vi "Update.vi"(8 "error in (no error)":errorcluster, 9 "Operation":enum16{"Get", "Set"}(ring), 11 "user event":refnum<user-event>) -> (0 "error out":errorcluster, 3 "user event (out)":refnum<user-event>)   [LabVIEW 2020, in "WebServiceImporter.lvlib" / "Main Panel.lvlib" / "Authentication.lvlib" / "Events.lvlib"]
uses:
  <vilib>/Platform/WebService/Main Panel/Pages/Authentication/Events/Events.lvlib
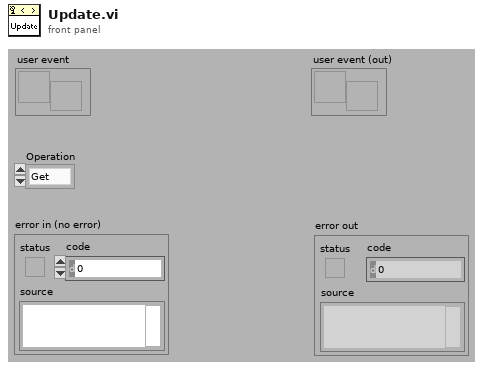
[diagram p1: front panel]
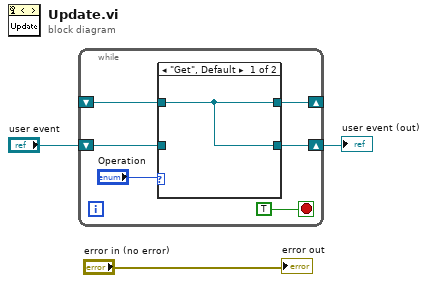
[diagram p0: block diagram]
diagram:
  n1 = while {
    shift-right: [w7] -> w1
    shift-left: "user event" -> [w8]
    shift-right: [w6] -> _
    shift-left: _ -> [w5]
    stop <- TRUE stop-if-true
    n2 = case shown="\"Get\", Default" "Operation" {
      tunnel: w8 -> [_ w11]
      tunnel: [w10 w11] -> w7
      tunnel: [w10 w11] -> w6
      tunnel: w5 -> [w10 _]
      frame "Get", Default {
      }
      frame "Set" {
      }
    }
  }
  "user event (out)" <- w1
  "error out" <- "error in (no error)"
